vi "EQ.vi"(8 "error in (no error)":errorcluster, 10 "Audio Block In":dbl[][](array[numeric]), 11 "Channel in":refnum<class "Channel.lvclass">) -> (0 "error out":errorcluster, 2 "Audio Block Out":dbl[][](array[numeric]))   [LabVIEW 2020, in "Channel.lvclass"]
doc: "Perform 3-band (low, mid, high) equalization of the audio data using Butterworth filters."
uses:
  Channel.lvclass
  Channel.lvclass/Channel.ctl
  <vilib>/Analysis/3filter.llb/Filter Passband Type.ctl
  Packed Libraries/Globals.lvlibp/Constants.vi
  <vilib>/Analysis/3filter.llb/Butterworth Filter (DBL).vi
  <vilib>/Analysis/3filter.llb/Bessel Filter.vi
  <vilib>/Analysis/3filter.llb/Bessel Filter (DBL).vi
  <vilib>/Analysis/NI_AALBase.lvlib
  Packed Libraries/Globals.lvlibp
  Libraries/User Interface/User Interface.lvlib
  Packed Libraries/Audio Processing.lvlibp
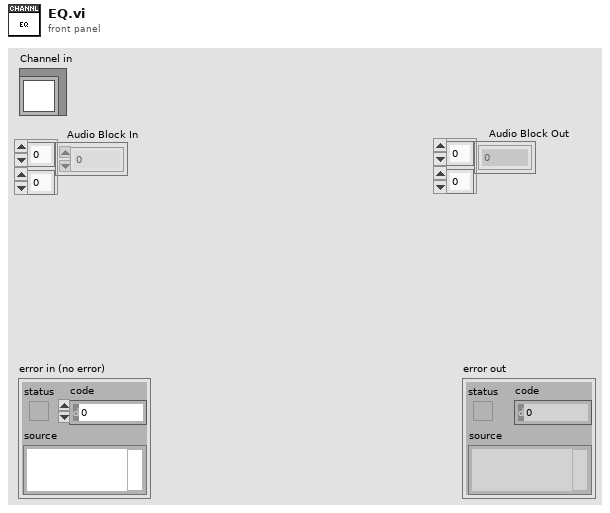
[diagram p1: front panel]
types:
  T1 = typedef "NI_AALBase.lvlib/Filter Passband Type.ctl" = enum32{"Lowpass", "Highpass", "Bandpass", "Bandstop"}
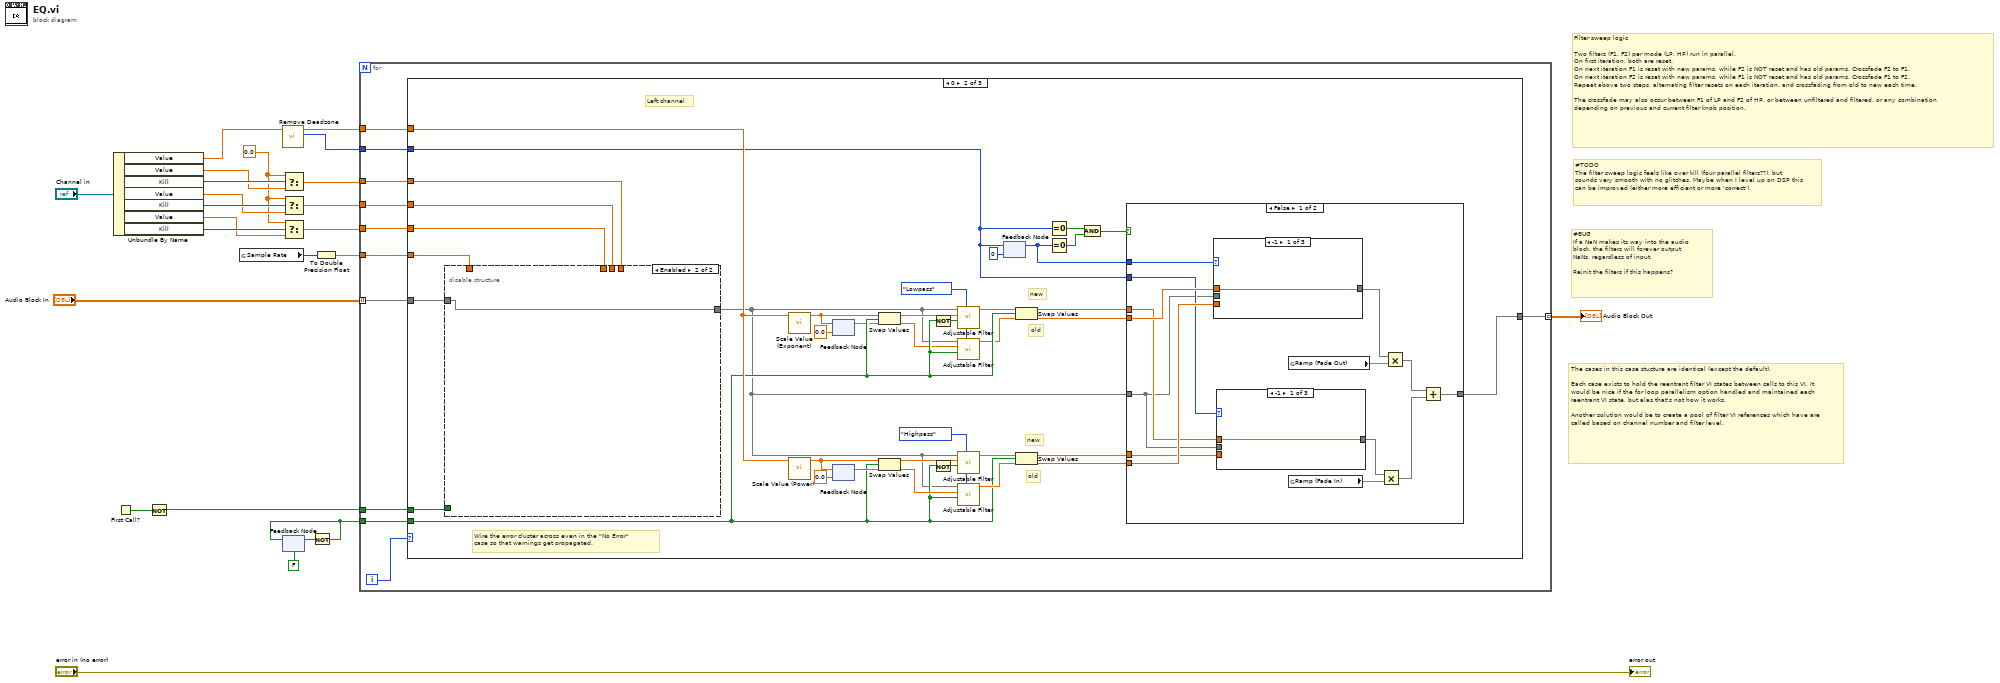
[diagram p0: block diagram]
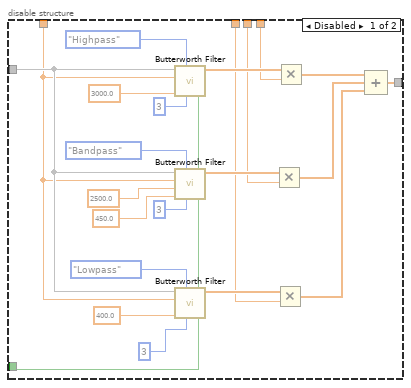
[diagram p3: hidden frame]
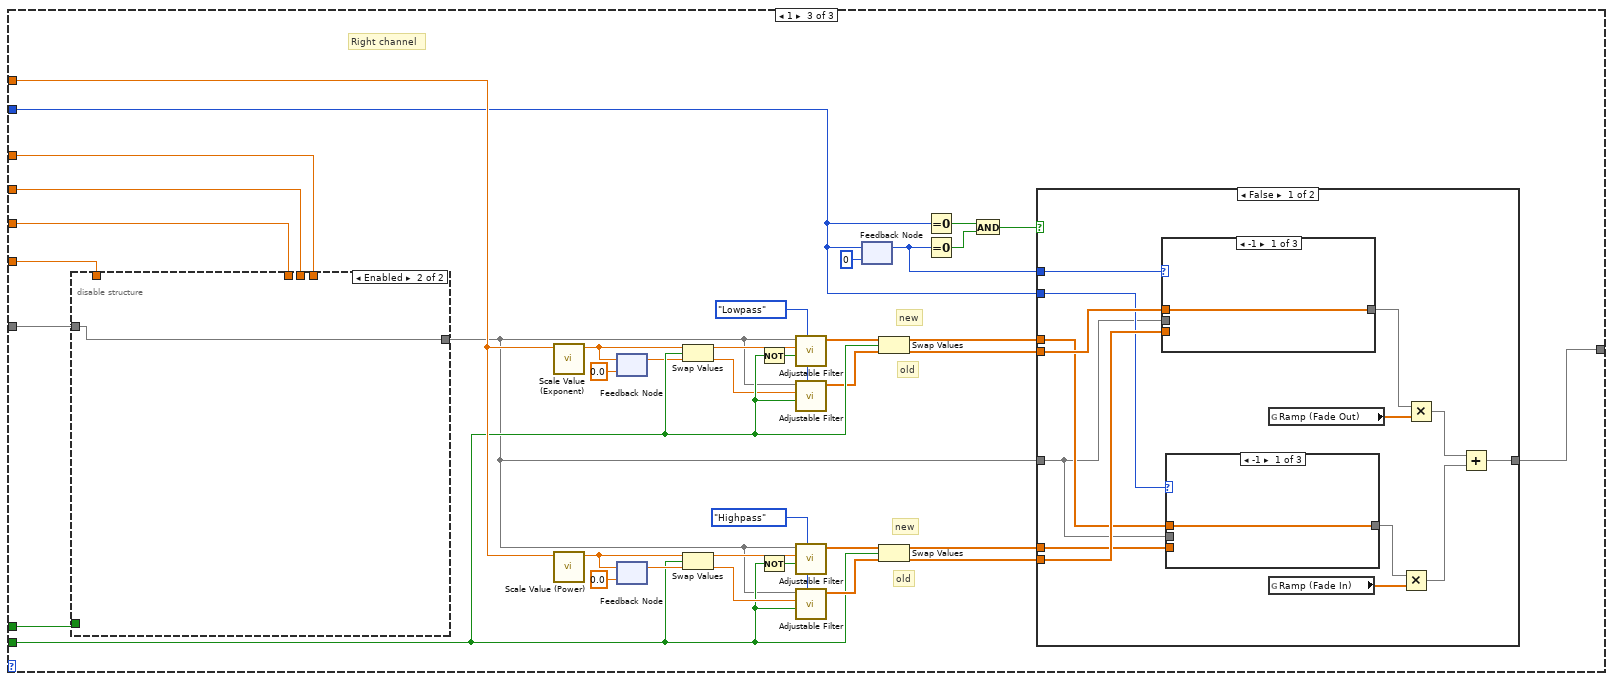
[diagram p9: hidden frame]
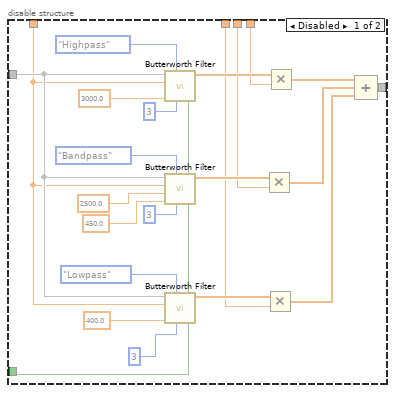
[diagram p10: hidden frame]
diagram:
  w17 = 0.0 ("t")
  # "Filter sweep logic\n\nTwo filters (F1, F2) per mode (LP, HP) run in parallel.\nOn first iteration, both are reset.\nOn next iteration F1 is reset with new params, while F2 is NOT reset and has old params. Crossfade F2 to F1.\nOn next iteration F2 is reset with new params, while F1 is NOT reset and has old params. Crossfade F1 to F2.\nRepeat above two steps, alternating filter resets on each iteration, and crossfading from old to new each time.\n\nThe crossfade may also occur between F1 of LP and F2 of HP, or between unfiltered and filtered, or any combination depending on previous and current filter knob position."
  # "#TODO\nThe filter sweep logic feels like over kill (four parallel filters??), but sounds very smooth with no glitches. Maybe when I level up on DSP this can be improved (either more efficient or more 'correct')."
  # "#BUG\nIf a NaN makes its way into the audio block, the filters will forever output NaNs, regardless of input.\n\nReinit the filters if this happens?"
  # "Wire the error cluster across even in the \"No Error\"\ncase so that warnings get propagated."
  # "The cases in this case stucture are identical (except the default).\n\nEach case exists to hold the reentrant filter VI states between calls to this VI. It would be nice if the for loop parallelism option handled and maintained each reentrant VI state, but alas that's not how it works.\n\nAnother solution would be to create a pool of filter VI references which have are called based on channel number and filter level."
  n1 = Unbundle By Name("Channel in") -> ("Value"=w6:dbl, "Value"=w20:dbl, "Kill"=w21:bool, "Value"=w18:dbl, "Kill"=w19:bool, "Value"=w15:dbl, "Kill"=w16:bool)
  n2 = First Call?() -> (First Call?: T/F=w11:bool)
  n3 = Not(x=w11) -> (.not. x?=w10:bool)
  n4 = global read "Constants.vi" "Sample Rate"() -> (w9:i32)
  n5 = call "Remove Deadzone.vi"("Value"=w6) -> ("Sign"=w4:i32, "Abs Value"=w5:dbl)  [unwired: 9 in]
  n6 = Select(t=w17, s=w21, f=w20) -> (s? t:f=w14:dbl)
  n7 = Select(t=w17, s=w19, f=w18) -> (s? t:f=w13:dbl)
  n8 = Select(t=w17, s=w16, f=w15) -> (s? t:f=w12:dbl)
  n9 = feedback #1(FALSE) -> (w2:bool)
  n10 = Not(x=w2) -> (.not. x?=w1:bool)
  n11 = feedback-in #1(w1) -> ()
  n12 = To Double Precision Float(number=w9) -> (double precision float=w8:dbl)
  n13 = for {
    tunnel: "Audio Block In" -> [w35] mode=indexing
    tunnel: w12 -> [w34]
    tunnel: w13 -> [w33]
    tunnel: w14 -> [w32]
    tunnel: [w26] -> w7 mode=indexing
    tunnel: w10 -> [w31]
    tunnel: w8 -> [w29]
    tunnel: w5 -> [w28]
    tunnel: w4 -> [w27]
    tunnel: w1 -> [w25]
    i -> [w30]
    n14 = case shown="0" w30 {
      tunnel: w35 -> [w36 w74 w157]
      tunnel: w34 -> [_ w73 w156]
      tunnel: w33 -> [_ w72 w155]
      tunnel: w32 -> [_ w71 w154]
      tunnel: [w36 w46 w129] -> w26
      tunnel: w31 -> [_ w70 w153]
      tunnel: w29 -> [_ w69 w152]
      tunnel: w28 -> [_ w60 w143]
      tunnel: w27 -> [_ w44 w127]
      tunnel: w25 -> [_ w59 w142]
      frame Default {
        # "Not expecting more than two channels, so pass them through unfiltered"
      }
      frame 0 {
        w51 = Filter_Passband_Type."Lowpass" ("Type (LP)")
        w61 = Filter_Passband_Type."Highpass" ("Type (LP)")
        # "old"
        # "new"
        # "old"
        # "new"
        # "Left channel"
        n15 = disable-structure shown="Enabled" {
          disable-tunnel: w74 -> [w86 w98]
          disable-tunnel: w73 -> [w85 _]
          disable-tunnel: w72 -> [w84 _]
          disable-tunnel: w71 -> [w83 _]
          disable-tunnel: w70 -> [w82 _]
          disable-tunnel: w69 -> [w76 _]
          disable-tunnel: [w75 w98] -> w47
          frame Disabled {
            n16 = call-poly <vilib>:"Butterworth Filter.vi"("init/cont (init:F)"=w82, "order"=3, "filter type"=Filter_Passband_Type."Highpass", "low cutoff freq: fl"=3000.0 ("high cutoff freq: fh"), "sampling freq: fs"=w76, "X"=w86) -> ("Filtered X"=w92:dbl[])  [unwired: 2 in, 1 out]
            n17 = call-poly <vilib>:"Butterworth Filter.vi"("init/cont (init:F)"=w82, "order"=3, "filter type"=Filter_Passband_Type."Bandpass", "low cutoff freq: fl"=450.0, "high cutoff freq: fh"=2500.0, "sampling freq: fs"=w76, "X"=w86) -> ("Filtered X"=w91:dbl[])  [unwired: 1 in, 1 out]
            n18 = call-poly <vilib>:"Butterworth Filter.vi"("init/cont (init:F)"=w82, "order"=3, "filter type"=Filter_Passband_Type."Lowpass", "low cutoff freq: fl"=400.0, "sampling freq: fs"=w76, "X"=w86) -> ("Filtered X"=w89:dbl[])  [unwired: 2 in, 1 out]
            n19 = Multiply(x=w91, y=w84) -> (x*y=w90:dbl[])
            n20 = Multiply(x=w89, y=w85) -> (x*y=w77:dbl[])
            n21 = Multiply(x=w92, y=w83) -> (x*y=w78:dbl[])
            n22 = Compound Arithmetic op=ADD(w78, w90, w77) -> (w75:dbl[])
          }
          frame Enabled {
          }
        }
        n23 = call "Scale Value (Exponent).vi"("Value"=w60) -> ("Scaled Value"=w57:dbl)  [unwired: 10 in]
        n24 = call "Scale Value (Power).vi"("Value"=w60) -> ("Scaled Value"=w67:dbl)  [unwired: 10 in]
        n25 = feedback #2(0.0 ("Scaled Value")) -> (w58:dbl)
        n26 = feedback-in #2(w57) -> ()
        n27 = feedback #3(0.0 ("Scaled Value")) -> (w68:dbl)
        n28 = feedback-in #3(w67) -> ()
        n29 = Swap Values(12:w57, 13:w59, 14:w58) -> (1:w56:dbl, 3:w55:dbl)
        n30 = Swap Values(12:w67, 13:w59, 14:w68) -> (1:w66:dbl, 3:w65:dbl)
        n31 = Not(x=w59) -> (.not. x?=w54:bool)
        n32 = Not(x=w59) -> (.not. x?=w64:bool)
        n33 = call "Adjustable Filter.vi"("Filter Type"=w51, "Reset Filter"=w54, "Frequency"=w56, "Audio Data"=w47) -> ("Filtered Audio Data"=w53:dbl[])  [unwired: 7 in]
        n34 = call "Adjustable Filter.vi"("Filter Type"=w51, "Reset Filter"=w59, "Frequency"=w55, "Audio Data"=w47) -> ("Filtered Audio Data"=w52:dbl[])  [unwired: 7 in]
        n35 = call "Adjustable Filter.vi"("Filter Type"=w61, "Reset Filter"=w64, "Frequency"=w66, "Audio Data"=w47) -> ("Filtered Audio Data"=w63:dbl[])  [unwired: 7 in]
        n36 = call "Adjustable Filter.vi"("Filter Type"=w61, "Reset Filter"=w59, "Frequency"=w65, "Audio Data"=w47) -> ("Filtered Audio Data"=w62:dbl[])  [unwired: 7 in]
        n37 = feedback #4(0 ("Sign")) -> (w45:i32)
        n38 = feedback-in #4(w44) -> ()
        n39 = Swap Values(12:w53, 13:w59, 14:w52) -> (1:w43:dbl[], 3:w42:dbl[])
        n40 = Swap Values(12:w63, 13:w59, 14:w62) -> (1:w41:dbl[], 3:w40:dbl[])
        n41 = Equal To 0?(x=w44) -> (x = 0?=w50:bool)
        n42 = Equal To 0?(x=w45) -> (x = 0?=w49:bool)
        n43 = And(x=w50, y=w49) -> (x .and. y?=w48:bool)
        n44 = case shown="False" w48 {
          tunnel: w47 -> [w105 w119]
          tunnel: [w99 w119] -> w46
          tunnel: w45 -> [w112 _]
          tunnel: w44 -> [w107 _]
          tunnel: w43 -> [w106 _]
          tunnel: w42 -> [w111 _]
          tunnel: w41 -> [w104 _]
          tunnel: w40 -> [w110 _]
          frame False {
            n45 = case shown="-1" w112 {
              tunnel: w111 -> [w116 _ _]
              tunnel: w105 -> [_ w117 _]
              tunnel: w110 -> [_ _ w118]
              tunnel: [w116 w117 w118] -> w108
              frame -1 {
              }
              frame 0, Default {
              }
              frame 1 {
              }
            }
            n46 = case shown="-1" w107 {
              tunnel: w106 -> [w113 _ _]
              tunnel: w105 -> [_ w114 _]
              tunnel: w104 -> [_ _ w115]
              tunnel: [w113 w114 w115] -> w102
              frame -1 {
              }
              frame 0, Default {
              }
              frame 1 {
              }
            }
            n47 = global read "Constants.vi" "Ramp (Fade Out)"() -> (w109:dbl[])
            n48 = global read "Constants.vi" "Ramp (Fade In)"() -> (w103:dbl[])
            n49 = Multiply(x=w102, y=w103) -> (x*y=w100:dbl[])
            n50 = Multiply(x=w108, y=w109) -> (x*y=w101:dbl[])
            n51 = Add(x=w101, y=w100) -> (x+y=w99:dbl[])
          }
          frame True {
          }
        }
      }
      frame 1 {
        w134 = Filter_Passband_Type."Lowpass" ("Type (LP)")
        w144 = Filter_Passband_Type."Highpass" ("Type (LP)")
        # "old"
        # "new"
        # "old"
        # "new"
        # "Right channel"
        n52 = disable-structure shown="Enabled" {
          disable-tunnel: w157 -> [w169 w181]
          disable-tunnel: w156 -> [w168 _]
          disable-tunnel: w155 -> [w167 _]
          disable-tunnel: w154 -> [w166 _]
          disable-tunnel: w153 -> [w165 _]
          disable-tunnel: w152 -> [w159 _]
          disable-tunnel: [w158 w181] -> w130
          frame Disabled {
            n53 = call-poly <vilib>:"Butterworth Filter.vi"("init/cont (init:F)"=w165, "order"=3, "filter type"=Filter_Passband_Type."Highpass", "low cutoff freq: fl"=3000.0 ("high cutoff freq: fh"), "sampling freq: fs"=w159, "X"=w169) -> ("Filtered X"=w175:dbl[])  [unwired: 2 in, 1 out]
            n54 = call-poly <vilib>:"Butterworth Filter.vi"("init/cont (init:F)"=w165, "order"=3, "filter type"=Filter_Passband_Type."Bandpass", "low cutoff freq: fl"=450.0, "high cutoff freq: fh"=2500.0, "sampling freq: fs"=w159, "X"=w169) -> ("Filtered X"=w174:dbl[])  [unwired: 1 in, 1 out]
            n55 = call-poly <vilib>:"Butterworth Filter.vi"("init/cont (init:F)"=w165, "order"=3, "filter type"=Filter_Passband_Type."Lowpass", "low cutoff freq: fl"=400.0, "sampling freq: fs"=w159, "X"=w169) -> ("Filtered X"=w172:dbl[])  [unwired: 2 in, 1 out]
            n56 = Multiply(x=w174, y=w167) -> (x*y=w173:dbl[])
            n57 = Multiply(x=w172, y=w168) -> (x*y=w160:dbl[])
            n58 = Multiply(x=w175, y=w166) -> (x*y=w161:dbl[])
            n59 = Compound Arithmetic op=ADD(w161, w173, w160) -> (w158:dbl[])
          }
          frame Enabled {
          }
        }
        n60 = call "Scale Value (Exponent).vi"("Value"=w143) -> ("Scaled Value"=w140:dbl)  [unwired: 10 in]
        n61 = call "Scale Value (Power).vi"("Value"=w143) -> ("Scaled Value"=w150:dbl)  [unwired: 10 in]
        n62 = feedback #5(0.0 ("Scaled Value")) -> (w141:dbl)
        n63 = feedback-in #5(w140) -> ()
        n64 = feedback #6(0.0 ("Scaled Value")) -> (w151:dbl)
        n65 = feedback-in #6(w150) -> ()
        n66 = Swap Values(12:w140, 13:w142, 14:w141) -> (1:w139:dbl, 3:w138:dbl)
        n67 = Swap Values(12:w150, 13:w142, 14:w151) -> (1:w149:dbl, 3:w148:dbl)
        n68 = Not(x=w142) -> (.not. x?=w137:bool)
        n69 = Not(x=w142) -> (.not. x?=w147:bool)
        n70 = call "Adjustable Filter.vi"("Filter Type"=w134, "Reset Filter"=w137, "Frequency"=w139, "Audio Data"=w130) -> ("Filtered Audio Data"=w136:dbl[])  [unwired: 7 in]
        n71 = call "Adjustable Filter.vi"("Filter Type"=w134, "Reset Filter"=w142, "Frequency"=w138, "Audio Data"=w130) -> ("Filtered Audio Data"=w135:dbl[])  [unwired: 7 in]
        n72 = call "Adjustable Filter.vi"("Filter Type"=w144, "Reset Filter"=w147, "Frequency"=w149, "Audio Data"=w130) -> ("Filtered Audio Data"=w146:dbl[])  [unwired: 7 in]
        n73 = call "Adjustable Filter.vi"("Filter Type"=w144, "Reset Filter"=w142, "Frequency"=w148, "Audio Data"=w130) -> ("Filtered Audio Data"=w145:dbl[])  [unwired: 7 in]
        n74 = feedback #7(0 ("Sign")) -> (w128:i32)
        n75 = feedback-in #7(w127) -> ()
        n76 = Swap Values(12:w136, 13:w142, 14:w135) -> (1:w126:dbl[], 3:w125:dbl[])
        n77 = Swap Values(12:w146, 13:w142, 14:w145) -> (1:w124:dbl[], 3:w123:dbl[])
        n78 = Equal To 0?(x=w127) -> (x = 0?=w133:bool)
        n79 = Equal To 0?(x=w128) -> (x = 0?=w132:bool)
        n80 = And(x=w133, y=w132) -> (x .and. y?=w131:bool)
        n81 = case shown="False" w131 {
          tunnel: w130 -> [w188 w202]
          tunnel: [w182 w202] -> w129
          tunnel: w128 -> [w195 _]
          tunnel: w127 -> [w190 _]
          tunnel: w126 -> [w189 _]
          tunnel: w125 -> [w194 _]
          tunnel: w124 -> [w187 _]
          tunnel: w123 -> [w193 _]
          frame False {
            n82 = case shown="-1" w195 {
              tunnel: w194 -> [w199 _ _]
              tunnel: w188 -> [_ w200 _]
              tunnel: w193 -> [_ _ w201]
              tunnel: [w199 w200 w201] -> w191
              frame -1 {
              }
              frame 0, Default {
              }
              frame 1 {
              }
            }
            n83 = case shown="-1" w190 {
              tunnel: w189 -> [w196 _ _]
              tunnel: w188 -> [_ w197 _]
              tunnel: w187 -> [_ _ w198]
              tunnel: [w196 w197 w198] -> w185
              frame -1 {
              }
              frame 0, Default {
              }
              frame 1 {
              }
            }
            n84 = global read "Constants.vi" "Ramp (Fade Out)"() -> (w192:dbl[])
            n85 = global read "Constants.vi" "Ramp (Fade In)"() -> (w186:dbl[])
            n86 = Multiply(x=w185, y=w186) -> (x*y=w183:dbl[])
            n87 = Multiply(x=w191, y=w192) -> (x*y=w184:dbl[])
            n88 = Add(x=w184, y=w183) -> (x+y=w182:dbl[])
          }
          frame True {
          }
        }
      }
    }
  }
  "Audio Block Out" <- w7
  "error out" <- "error in (no error)"
